vi "pruebaspexx.vi"() -> ()   [LabVIEW 2016]
panel:
  out "lamda":dbl
  in  "paso":dbl
  in  "fin":dbl
  in  "inicio":dbl
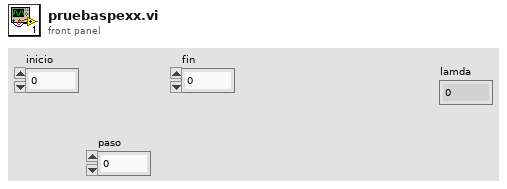
[diagram p1: front panel]
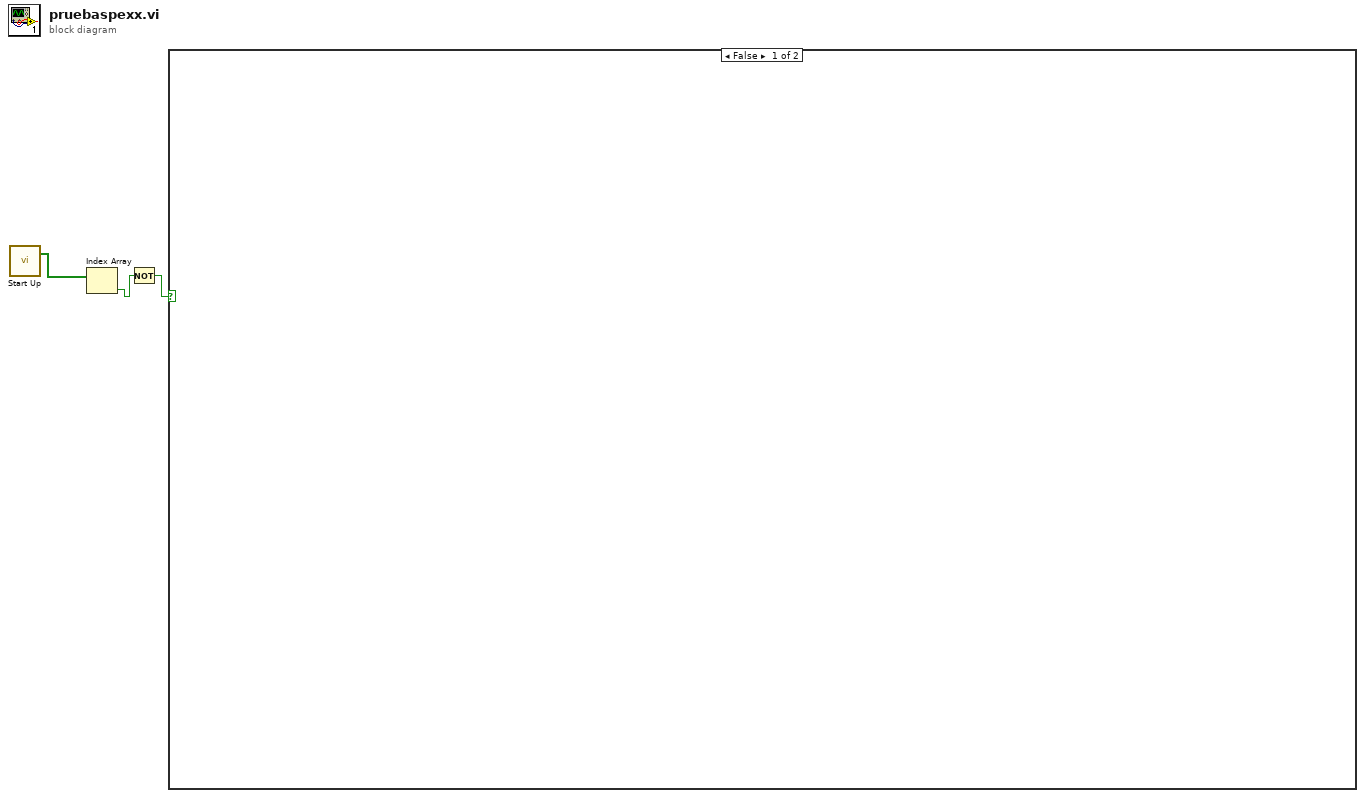
[diagram p0: block diagram]
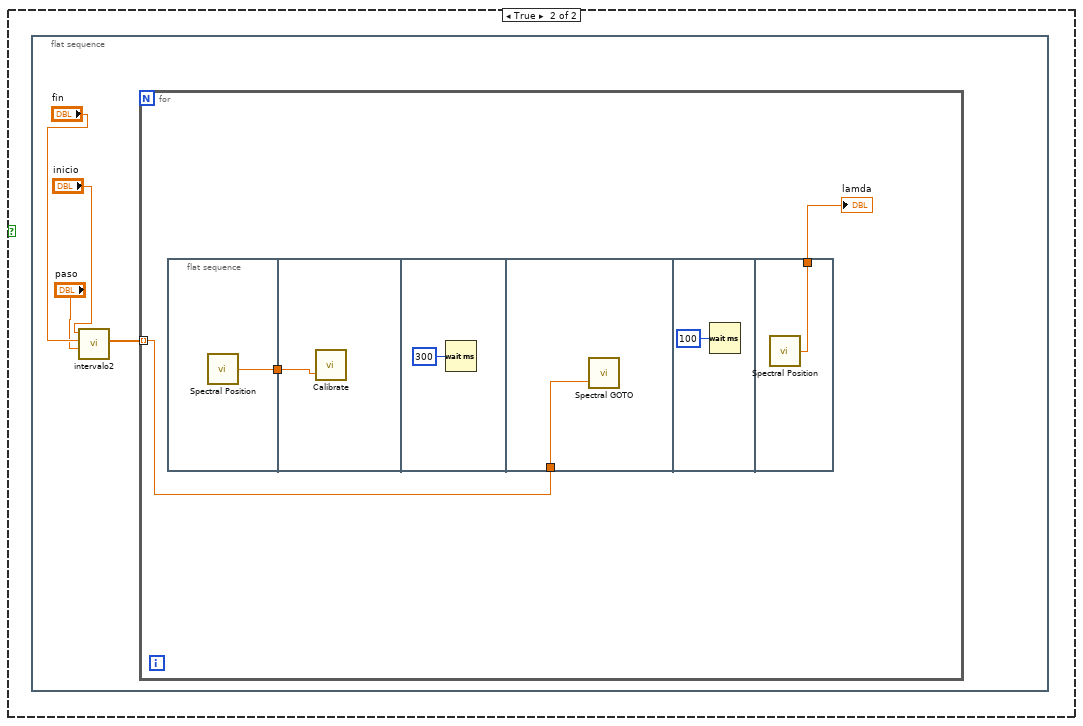
[diagram p2: hidden frame]
diagram:
  n1 = call "Start Up.VI"() -> ("Error List"=w3:bool[])  [unwired: 1 in, 1 out]
  n2 = Index Array(array=w3) -> (element=w2:bool)  [unwired: 1 in]
  n3 = Not(x=w2) -> (.not. x?=w1:bool)
  n4 = case shown="False" w1 {
    frame False {
    }
    frame True {
      n5 = flat-sequence {
        frame #0 {
          n6 = call "intervalo2.vi"("incremento"="paso", "fin"="fin", "inicio"="inicio") -> ("Array"=w7:dbl[])  [unwired: 8 in]
          n7 = for {
            tunnel: w7 -> [w9] mode=indexing
            n8 = flat-sequence {
              tunnel: [w11] -> w10
              tunnel: w10 -> [w12]
              tunnel: w9 -> [w14]
              tunnel: [w16] -> w8
              frame #0 {
                n9 = call "Spectral Position.VI"() -> ("Present Position"=w11:dbl)  [unwired: 1 in, 2 out]
              }
              frame #1 {
                n10 = call "Calibrate.VI"("Counter Position"=w12) -> ()  [unwired: 1 in, 3 out]
              }
              frame #2 {
                n11 = Wait (ms)(milliseconds to wait=u32 300) -> ()  [unwired: 1 out]
              }
              frame #3 {
                n12 = call "Spectral GOTO.VI"("Target Position"=w14) -> ()  [unwired: 1 in, 3 out]
              }
              frame #4 {
                n13 = Wait (ms)(milliseconds to wait=u32 100) -> ()  [unwired: 1 out]
              }
              frame #5 {
                n14 = call "Spectral Position.VI"() -> ("Present Position"=w16:dbl)  [unwired: 1 in, 2 out]
              }
            }
            "lamda" <- w8
          }
        }
      }
    }
  }
